vi "dfd_Multirate Filter Design.vi"(5 "method":u16(ring)=2 items=["Kaiser Window", "Dolph-Chebyshev Window", "Equi-Ripple", "Positive Equi-Ripple"], 6 "band option":enum16{"Normal", "Nyquist", "Alias free"}(ring), 7 "#band":i32=2, 8 "error IO":errorcluster, 10 "roll off":dbl=2.0, 11 "order":i32=20) -> (0 "error out":errorcluster, 2 "order out":i32, 3 "h out":dbl[](array[numeric]))   [LabVIEW 2017, in "NI_DigFilter_Process.lvlib"]
uses:
  <vilib>/addons/Digital Filter Design/NI_DigFilter_Process.lvlib
  <vilib>/addons/Digital Filter Design/_REMEZ.llb/remez_fir filter type.ctl
  <vilib>/addons/Digital Filter Design/NI_DigFilter_Design.lvlib
  <vilib>/addons/Digital Filter Design/NI_DigFilterLicensed.lvlib
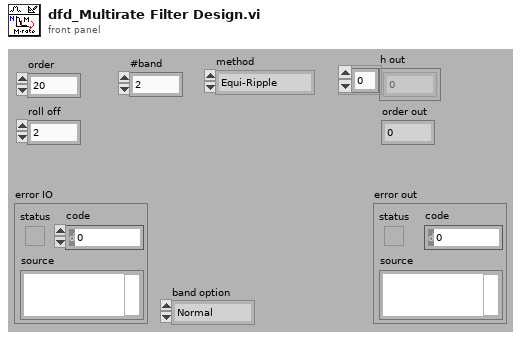
[diagram p1: front panel]
types:
  T1 = enum16{"Lowpass", "Highpass", "Bandpass", "Bandstop"}
  T2 = typedef "NI_DigFilterLicensed.lvlib/remez_fir filter type.ctl" = enum32{"Symmetric", "Antisymmetric", "Differentiator", "Hilbert", "Minimum Phase", "Maximum Phase"}
  T3 = typedef "NI_DigFilterLicensed.lvlib/DFD Adv Band Spec.ctl" = cluster{"band specification":cluster{"freq":dbl, "amplitude":dbl, "weight":dbl}[], "ripple constraint":dbl}
  T4 = typedef "remez_band specification.ctl" = T5[]
  T5 = typedef "remez_single band description.ctl" = cluster{"points":cluster{"f":dbl, "A":dbl, "W":dbl, "forced gain?":bool}[], "band weight":dbl, "constraint":dbl, "ripple idx":i32, "in band weight option":enum16{"ignore", "linear interpolation", "const amplitude %"}}
  T6 = typedef "remez_fir order and types.ctl" = cluster{"# of taps":i32, "filter type":T2, "minimum order":enum32{"user defined", "minEven", "minOdd"}}
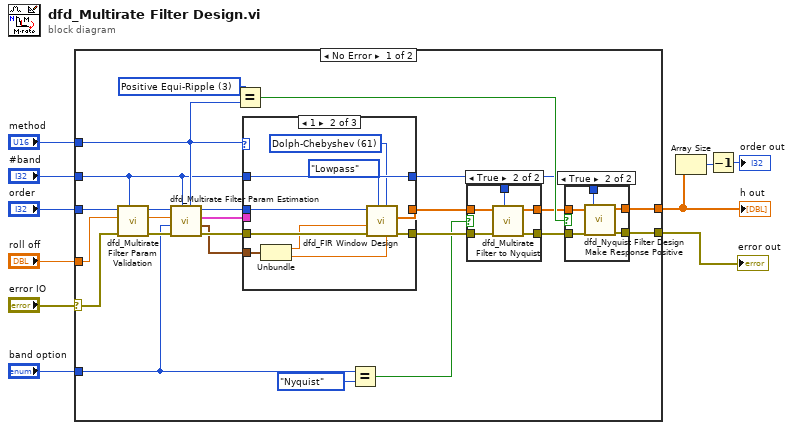
[diagram p0: block diagram]
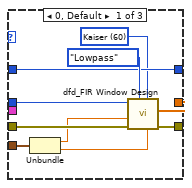
[diagram p4: hidden frame]
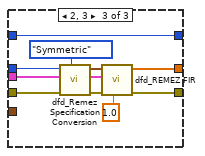
[diagram p5: hidden frame]
diagram:
  n1 = case shown="No Error" "error IO" {
    selector: "error IO" -> [w18 w80]
    tunnel: "method" -> [w33 _]
    tunnel: [w31 w80] -> w9
    tunnel: "#band" -> [w28 _]
    tunnel: "roll off" -> [w24 _]
    tunnel: "order" -> [w23 _]
    tunnel: [w19 _] -> w4
    tunnel: "band option" -> [w15 _]
    frame No Error {
      w11 = u16 3 items=["Kaiser Window", "Dolph-Chebyshev Window", "Equi-Ripple", "Positive Equi-Ripple"] ("method")
      n2 = call <vilib>:"dfd_Multirate Filter Param Validation.vi"("multirate factor"=w28, "error in (no error)"=w18, "roll off"=w24, "order"=w23) -> ("error out"=w25:errorcluster, "dup roll off"=w27:dbl, "dup order"=w26:i32)  [unwired: 2 in, 3 out]
      n3 = call <vilib>:"dfd_Multirate Filter Param Estimation.vi"("method"=w33, "multirate factor"=w28, "error in (no error)"=w25, "option"=w15, "roll off"=w27, "order"=w26) -> ("error out"=w22:errorcluster, "window param"=w17:cluster{"low cutoff freq: fl":dbl, "param":dbl}, "band parameters"=w20:T3[], "new order"=w21:i32)  [unwired: 2 out]
      n4 = Equal?(x=w11, y=w33) -> (x = y?=w34:bool)
      n5 = case shown="1" w33 {
        tunnel: [w54 w64 w77] -> w12
        tunnel: [w53 w63 w76] -> w16
        tunnel: w20 -> [_ _ w73]
        tunnel: w21 -> [w57 w67 w72]
        tunnel: w22 -> [w56 w66 w74]
        tunnel: w28 -> [w55 w65 w78]
        tunnel: [w55 w65 w78] -> w32
        tunnel: w17 -> [w52 w62 _]
        frame 0, Default {
          w49 = u16 60 items=["None"=0, "Hanning"=1, "Hamming"=2, "Blackman-Harris"=3, "Exact Blackman"=4, "Blackman"=5, "Flat Top"=6, "4 Term B-Harris"=7, "7 Term B-Harris"=8, "Low Sidelobe"=9, "Triangular"=30, "Kaiser"=60, "Dolph-Chebyshev"=61] ("window")
          n6 = Unbundle(w52) -> ("low cutoff freq: fl"=w51:dbl, "param"=w50:dbl)
          n7 = call <vilib>:"dfd_FIR Window Design.vi"("param"=w50, "window"=w49, "filter type"=T1."Lowpass", "error in (no error)"=w56, "low cutoff freq: fl"=w51, "order"=w57) -> ("error out"=w53:errorcluster, "h"=w54:dbl[])  [unwired: 2 in, 2 out]
        }
        frame 1 {
          w59 = u16 61 items=["None"=0, "Hanning"=1, "Hamming"=2, "Blackman-Harris"=3, "Exact Blackman"=4, "Blackman"=5, "Flat Top"=6, "4 Term B-Harris"=7, "7 Term B-Harris"=8, "Low Sidelobe"=9, "Triangular"=30, "Kaiser"=60, "Dolph-Chebyshev"=61] ("window")
          n8 = Unbundle(w62) -> ("low cutoff freq: fl"=w61:dbl, "param"=w60:dbl)
          n9 = call <vilib>:"dfd_FIR Window Design.vi"("param"=w60, "window"=w59, "filter type"=T1."Lowpass", "error in (no error)"=w66, "low cutoff freq: fl"=w61, "order"=w67) -> ("error out"=w63:errorcluster, "h"=w64:dbl[])  [unwired: 2 in, 2 out]
        }
        frame 2, 3 {
          n10 = call <vilib>:"dfd_Remez Specification Conversion.vi"("phase option"=remez_fir_filter_type."Symmetric" ("filter type"), "error in (no error)"=w74, "band parameters"=w73, "order"=w72) -> ("error out"=w71:errorcluster, "band specification"=w70:T4, "order and type"=w69:T6)  [unwired: 2 in, 3 out]
          n11 = call <vilib>:"dfd_REMEZ FIR.vi"("fs"=1.0 ("fs [Hz]"), "error in (no error)"=w71, "band specification"=w70, "order and type"=w69) -> ("error out"=w76:errorcluster, "h"=w77:dbl[])  [unwired: 1 in, 5 out]
        }
      }
      n12 = Equal?(x=w15, y=enum16{"Normal", "Nyquist", "Alias free"}."Nyquist") -> (x = y?=w13:bool)
      n13 = case shown="True" w13 {
        tunnel: w32 -> [_ w41]
        tunnel: [w36 w40] -> w30
        tunnel: [w35 w39] -> w29
        tunnel: w16 -> [w35 w38]
        tunnel: w12 -> [w36 w37]
        frame False {
        }
        frame True {
          n14 = call <vilib>:"dfd_Multirate Filter to Nyquist.vi"("#band"=w41, "error in (no error)"=w38, "h in"=w37) -> ("error out"=w39:errorcluster, "h out"=w40:dbl[])  [unwired: 4 in, 3 out]
        }
      }
      n15 = case shown="True" w34 {
        tunnel: w29 -> [w42 w48]
        tunnel: w30 -> [w43 w47]
        tunnel: [w43 w46] -> w19
        tunnel: [w42 w45] -> w31
        tunnel: w32 -> [_ w44]
        frame False {
        }
        frame True {
          n16 = call <vilib>:"dfd_Nyquist Filter Design Make Response Positive.vi"("#band"=w44, "error in (no error)"=w48, "h in"=w47) -> ("error out"=w45:errorcluster, "h out"=w46:dbl[])  [unwired: 2 in, 5 out]
        }
      }
    }
    frame Error {
    }
  }
  "error out" <- w9
  "h out" <- w4
  n17 = Array Size(array=w4) -> (size(s)=w5:i32)
  n18 = Decrement(x=w5) -> (x-1=→"order out":i32)
